vi "Error Dialog.vi"(8 "error in (no error)":errorcluster, 9 "Show Dialog? (T)":bool=TRUE) -> (0 "error out":errorcluster, 1 "message":string)   [LabVIEW 2019, in "Script.lvlib"]
doc: "This VI replaces the \"Simple Error Handler.vi\" to remove the vi.lib dependencies.\n\nCreated By: Ryan Pacini"
uses:
  Script.lvlib
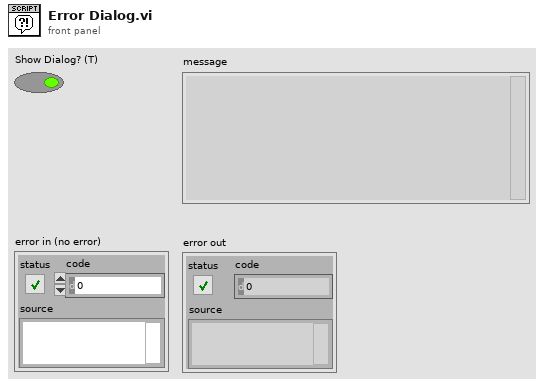
[diagram p1: front panel]
types:
  T1 = cluster{"Error %d occurred at %s":string, "Warning %d occurred at %s":string, "Possible reasons: %s":string, "Error not listed":string, "GetCommError x%lx":string, "Continue":string, "Stop":string, "an unidentified location":string, "No Error":string, "Help":string}
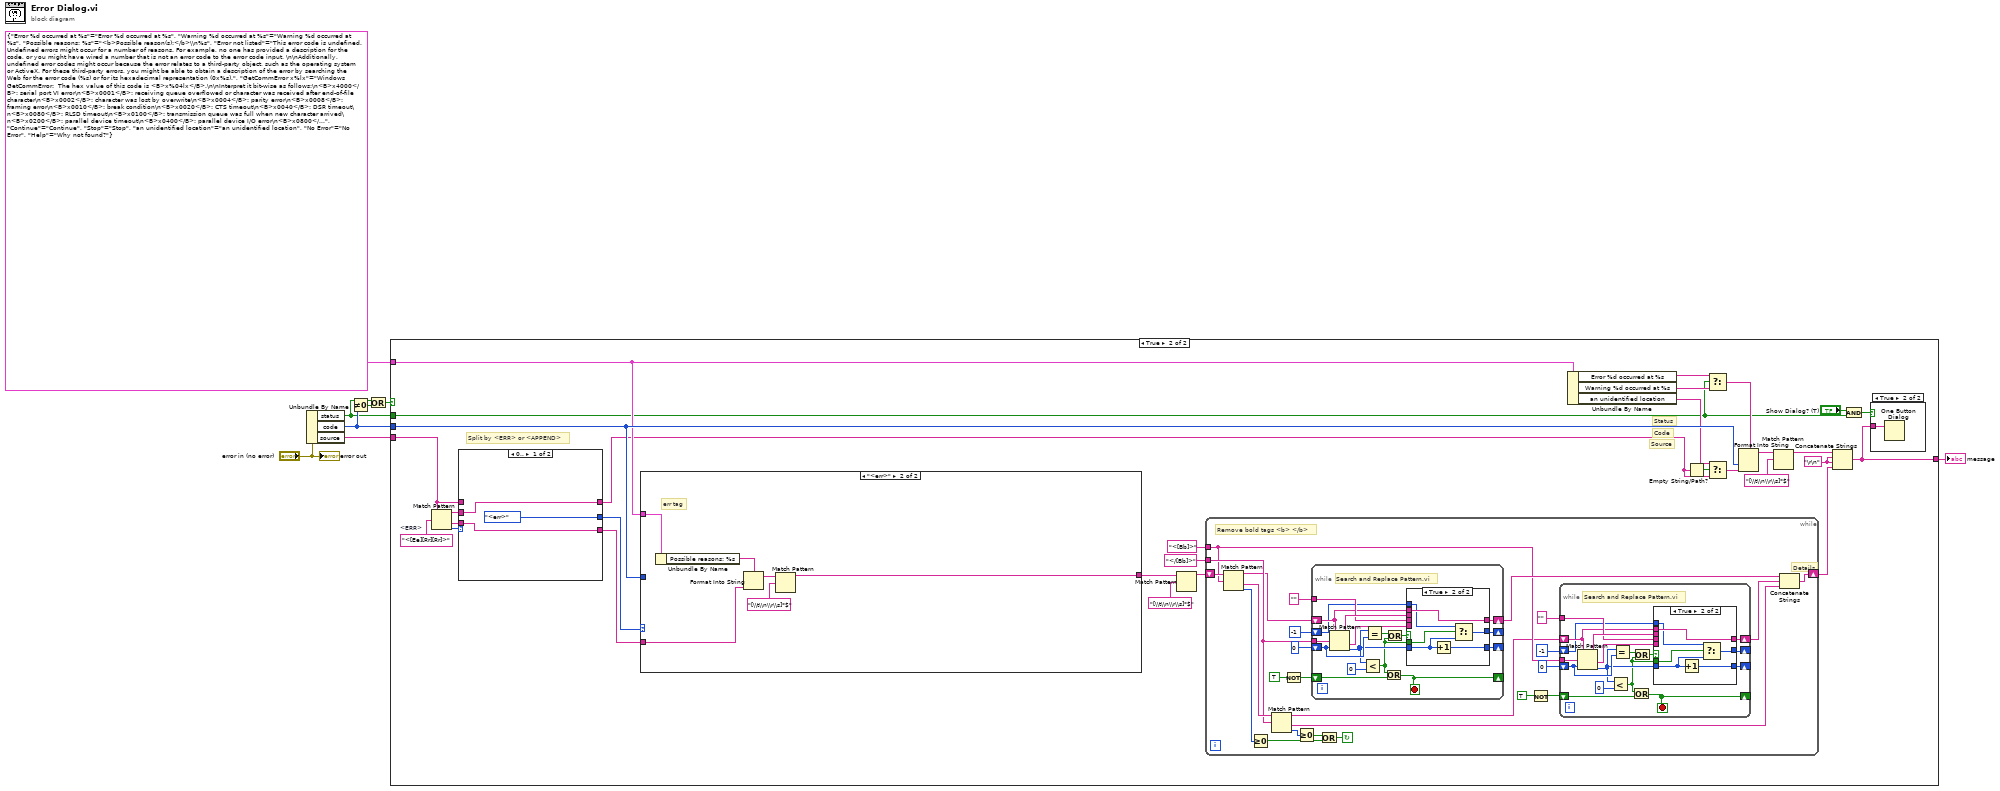
[diagram p0: block diagram]
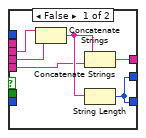
[diagram p3: hidden frame]
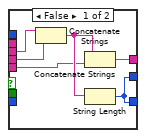
[diagram p4: hidden frame]
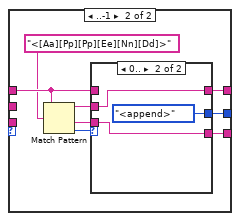
[diagram p5: hidden frame]
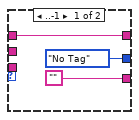
[diagram p6: hidden frame]
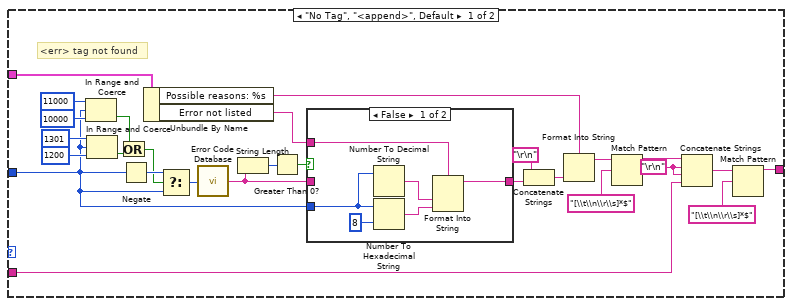
[diagram p7: hidden frame]
diagram:
  n1 = Unbundle By Name("error in (no error)") -> ("status"=w4:bool, "code"=w5:i32, "source"=w3:string)
  n2 = Not Equal To 0?(x=w5) -> (x != 0?=w7:bool)
  n3 = Or(x=w4, y=w7) -> (x .or. y?=w6:bool)
  n4 = case shown="True" w6 {
    tunnel: [_ w17] -> w8
    tunnel: w4 -> [_ w15]
    tunnel: w3 -> [_ w29]
    tunnel: w5 -> [_ w37]
    tunnel: T1 {"Error %d occurred at %s"="Error %d occurred at %s", "Warning %d occurred at %s"="Warning %d occurred at %s", "Possible reasons: %s"="<b>Possible reason(s):</b>\\n%s", "Error not listed"="This error code is undefined. Undefined errors might occur for a number of reasons. For example, no one has provided a description for the code, or you might have wired a number that is not an error code to the error code input. \n\nAdditionally, undefined error codes might occur because the error relates to a third-party object, such as the operating system or ActiveX. For these third-party errors, you might be able to obtain a description of the error by searching the Web for the error code (%s) or for its hexadecimal representation (0x%s).", "GetCommError x%lx"="Windows GetCommError:  The hex value of this code is <B>x%04lx</B>.\n\nInterpret it bit-wise as follows:\n<B>x4000</B>: serial port VI error\n<B>x0001</B>: receiving queue overflowed or character was received after end-of-file character\n<B>x0002</B>: character was lost by overwrite\n<B>x0004</B>: parity error\n<B>x0008</B>: framing error\n<B>x0010</B>: break condition\n<B>x0020</B>: CTS timeout\n<B>x0040</B>: DSR timeout\n<B>x0080</B>: RLSD timeout\n<B>x0100</B>: transmission queue was full when new character arrived\n<B>x0200</B>: parallel device timeout\n<B>x0400</B>: parallel device I/O error\n<B>x0800</B>: parallel device not selected\n<B>x1000</B>: parallel device out of paper\n<B>x8000</B>: requested mode is  not supported or the idComDev parameter is invalid.", "Continue"="Continue", "Stop"="Stop", "an unidentified location"="an unidentified location", "No Error"="No Error", "Help"="Why not found?"} ("prompts") -> [_ w31]
    frame False {
    }
    frame True {
      w19 = "\r\n"
      w32 = "<[Ee][Rr][Rr]>"  # <ERR>
      # "Code"
      # "Status"
      # "Details"
      # "Source"
      # "Split by <ERR> or <APPEND>"
      n5 = Match Pattern(string=w29, regular expression=w32) -> (before substring=w33:string, after substring=w34:string, offset past match=w35:i32)  [unwired: 1 in, 1 out]
      n6 = case shown="0.." w35 {
        tunnel: w33 -> [w123 _]
        tunnel: w34 -> [w124 _]
        tunnel: [w124 w131] -> w38
        tunnel: [w123 w129] -> w30
        tunnel: [enum16{"No Tag", "<err>", "<append>"}."<err>" ("Tag Found?") w128] -> w36
        tunnel: w29 -> [_ w127]
        frame 0.. {
        }
        frame ..-1 {
          n7 = Match Pattern(string=w127, regular expression="<[Aa][Pp][Pp][Ee][Nn][Dd]>") -> (before substring=w132:string, after substring=w130:string, offset past match=w126:i32)  [unwired: 1 in, 1 out]
          n8 = case shown="0.." w126 {
            tunnel: w132 -> [_ w137]
            tunnel: ["" w138] -> w131
            tunnel: w130 -> [_ w138]
            tunnel: [w135 w137] -> w129
            tunnel: [enum16{"No Tag", "<err>", "<append>"}."No Tag" ("Tag Found?") enum16{"No Tag", "<err>", "<append>"}."<append>" ("Tag Found?")] -> w128
            tunnel: w127 -> [w135 _]
            frame ..-1 {
            }
            frame 0.. {
            }
          }
        }
      }
      n9 = case shown="\"<err>\"" w36 {
        tunnel: [w152 w177] -> w10
        tunnel: w37 -> [w150 _]
        tunnel: w38 -> [w153 w176]
        tunnel: w31 -> [w149 w175]
        frame "No Tag", "<append>", Default {
          w139 = "\r\n" ("End of Line Constant")
          # "<err> tag not found"
          n10 = In Range and Coerce(upper limit=11000, x=w150, lower limit=10000) -> (In Range?=w160:bool)  [unwired: 1 out]
          n11 = In Range and Coerce(upper limit=1301, x=w150, lower limit=1200) -> (In Range?=w161:bool)  [unwired: 1 out]
          n12 = Or(x=w160, y=w161) -> (x .or. y?=w159:bool)
          n13 = Negate(x=w150) -> (-x=w163:i32)
          n14 = Unbundle By Name(w149) -> ("Possible reasons: %s"=w147:string, "Error not listed"=w148:string)
          n15 = Select(t=w163, s=w159, f=w150) -> (s? t:f=w151:i32)
          n16 = call <vilib>:"Error Code Database.vi"("Error Code"=w151) -> ("Error Text"=w155:string)
          n17 = String Length(string=w155) -> (length=w157:i32)
          n18 = Greater Than 0?(x=w157) -> (x > 0?=w156:bool)
          n19 = case shown="False" w156 {
            tunnel: [w170 w172] -> w154
            tunnel: w155 -> [_ w172]
            tunnel: w150 -> [w167 _]
            tunnel: w148 -> [w166 _]
            frame False {
              n20 = Number To Decimal String(number=w167) -> (decimal integer string=w168:string)  [unwired: 1 in]
              n21 = Number To Hexadecimal String(1:i16 8 ("width (-)"), 2:w167) -> (0:w169:string)
              n22 = Format Into String(format string=w166, w168, w169) -> (resulting string=w170:string)  [unwired: 2 in, 1 out]
            }
            frame True {
              # "Error code text found"
            }
          }
          n23 = Concatenate Strings("\r\n" ("End of Line Constant"), w154) -> (w146:string)
          n24 = Format Into String(format string=w147, w146) -> (resulting string=w143:string)  [unwired: 2 in, 1 out]
          n25 = Match Pattern(string=w143, regular expression="[\\t\\n\\r\\s]*$") -> (before substring=w142:string)  [unwired: 1 in, 3 out]
          n26 = Concatenate Strings(w142, w139, w139, w153) -> (w140:string)
          n27 = Match Pattern(string=w140, regular expression="[\\t\\n\\r\\s]*$") -> (before substring=w152:string)  [unwired: 1 in, 3 out]
        }
        frame "<err>" {
          # "err tag"
          n28 = Unbundle By Name(w175) -> ("Possible reasons: %s"=w174:string)
          n29 = Format Into String(format string=w174, w176) -> (resulting string=w178:string)  [unwired: 2 in, 1 out]
          n30 = Match Pattern(string=w178, regular expression="[\\t\\n\\r\\s]*$") -> (before substring=w177:string)  [unwired: 1 in, 3 out]
        }
      }
      n31 = Match Pattern(string=w10, regular expression="[\\t\\n\\r\\s]*$") -> (before substring=w11:string)  [unwired: 1 in, 3 out]
      n32 = while {
        shift-right: [w60] -> w9
        shift-left: w11 -> [w62]
        tunnel: "<[Bb]>" ("don't translate!") -> [w41]
        tunnel: "</[Bb]>" ("don't translate!") -> [w49]
        stop <- w55 continue-if-true
        # "Remove bold tags <b> </b>"
        n33 = Match Pattern(string=w62, regular expression=w41) -> (before substring=w47:string, after substring=w63:string, offset past match=w59:i32)  [unwired: 1 in, 1 out]
        n34 = Greater Or Equal To 0?(x=w59) -> (x >= 0?=w56:bool)
        n35 = Match Pattern(string=w63, regular expression=w49) -> (before substring=w40:string, after substring=w61:string, offset past match=w58:i32)  [unwired: 1 in, 1 out]
        n36 = Not(x=TRUE ("replace all? (F)")) -> (.not. x?=w54:bool)
        n37 = Greater Or Equal To 0?(x=w58) -> (x >= 0?=w57:bool)
        n38 = while {
          shift-right: [w74] -> _
          shift-left: w54 -> [w75]
          shift-right: [w72] -> _
          shift-left: 0 ("offset (0)") -> [w68]
          shift-right: [w76] -> w48
          shift-left: w47 -> [w73]
          tunnel: w49 -> [w80]
          tunnel: "" ("replace string (\"\")") -> [w77]
          shift-right: [w66] -> _
          shift-left: -1 -> [w65]
          stop <- w74 stop-if-true
          # "Search and Replace Pattern.vi"
          n39 = Match Pattern(string=w73, regular expression=w80, offset (0)=w68) -> (before substring=w79:string, after substring=w78:string, offset past match=w67:i32)  [unwired: 1 out]
          n40 = Less?(x=w67, y=0) -> (x < y?=w64:bool)
          n41 = Equal?(x=w67, y=w68) -> (x = y?=w69:bool)
          n42 = Or(x=w64, y=w75) -> (x .or. y?=w74:bool)
          n43 = Or(x=w69, y=w64) -> (x .or. y?=w70:bool)
          n44 = case shown="True" w70 {
            tunnel: w79 -> [w85 _]
            tunnel: w78 -> [w82 _]
            tunnel: w77 -> [w84 _]
            tunnel: [w86 w92] -> w76
            tunnel: w73 -> [_ w92]
            tunnel: [w81 w91] -> w72
            tunnel: w67 -> [_ w88]
            tunnel: [w81 w87] -> w66
            tunnel: w65 -> [_ w89]
            tunnel: w64 -> [_ w90]
            frame False {
              n45 = Concatenate Strings(w85, w84) -> (w83:string)
              n46 = Concatenate Strings(w83, w82) -> (w86:string)
              n47 = String Length(string=w83) -> (length=w81:i32)
            }
            frame True {
              n48 = Increment(x=w88) -> (x+1=w91:i32)
              n49 = Select(t=w89, s=w90, f=w88) -> (s? t:f=w87:i32)
            }
          }
        }
        n50 = Or(x=w57, y=w56) -> (x .or. y?=w55:bool)
        n51 = Not(x=TRUE ("replace all? (F)")) -> (.not. x?=w42:bool)
        n52 = while {
          shift-right: [w103] -> _
          shift-left: w42 -> [w104]
          shift-right: [w101] -> _
          shift-left: 0 ("offset (0)") -> [w97]
          shift-right: [w105] -> w39
          shift-left: w40 -> [w102]
          tunnel: w41 -> [w109]
          tunnel: "" ("replace string (\"\")") -> [w106]
          shift-right: [w95] -> _
          shift-left: -1 -> [w94]
          stop <- w103 stop-if-true
          # "Search and Replace Pattern.vi"
          n53 = Match Pattern(string=w102, regular expression=w109, offset (0)=w97) -> (before substring=w108:string, after substring=w107:string, offset past match=w96:i32)  [unwired: 1 out]
          n54 = Less?(x=w96, y=0) -> (x < y?=w93:bool)
          n55 = Equal?(x=w96, y=w97) -> (x = y?=w98:bool)
          n56 = Or(x=w93, y=w104) -> (x .or. y?=w103:bool)
          n57 = Or(x=w98, y=w93) -> (x .or. y?=w99:bool)
          n58 = case shown="True" w99 {
            tunnel: w108 -> [w114 _]
            tunnel: w107 -> [w111 _]
            tunnel: w106 -> [w113 _]
            tunnel: [w115 w121] -> w105
            tunnel: w102 -> [_ w121]
            tunnel: [w110 w120] -> w101
            tunnel: w96 -> [_ w117]
            tunnel: [w110 w116] -> w95
            tunnel: w94 -> [_ w118]
            tunnel: w93 -> [_ w119]
            frame False {
              n59 = Concatenate Strings(w114, w113) -> (w112:string)
              n60 = Concatenate Strings(w112, w111) -> (w115:string)
              n61 = String Length(string=w112) -> (length=w110:i32)
            }
            frame True {
              n62 = Increment(x=w117) -> (x+1=w120:i32)
              n63 = Select(t=w118, s=w119, f=w117) -> (s? t:f=w116:i32)
            }
          }
        }
        n64 = Concatenate Strings(w48, w39, w61) -> (w60:string)
      }
      n65 = Unbundle By Name(w31) -> ("Error %d occurred at %s"=w23:string, "Warning %d occurred at %s"=w27:string, "an unidentified location"=w24:string)
      n66 = Empty String/Path?(string/path=w30) -> (empty?=w28:bool)
      n67 = Select(t=w23, s=w15, f=w27) -> (s? t:f=w26:string)
      n68 = Select(t=w24, s=w28, f=w30) -> (s? t:f=w25:string)
      n69 = Format Into String(format string=w26, w37, w25) -> (resulting string=w21:string)  [unwired: 2 in, 1 out]
      n70 = Match Pattern(string=w21, regular expression="[\\t\\n\\r\\s]*$") -> (before substring=w20:string)  [unwired: 1 in, 3 out]
      n71 = Concatenate Strings(w20, w19, w19, w9) -> (w17:string)
      n72 = And(x="Show Dialog? (T)", y=w15) -> (x .and. y?=w16:bool)
      n73 = case shown="True" w16 {
        tunnel: w17 -> [_ w179]
        frame False {
        }
        frame True {
          n74 = One Button Dialog(message=w179) -> ()  [unwired: 1 in, 1 out]
        }
      }
    }
  }
  "message" <- w8
  "error out" <- "error in (no error)"
